vi "Init Hardware.vi"(8 "error in (no error)":errorcluster, 11 "Fluke 1586A Driver in":refnum<class "Fluke 1586A Driver.lvclass">) -> (0 "error out":errorcluster, 3 "Fluke 1586A Driver out":refnum<class "Fluke 1586A Driver.lvclass">)   [LabVIEW 2024, in "Fluke 1586A Driver.lvclass"]
uses:
  Fluke 1586A Driver.lvclass
  Instrument Driver/Instrument Driver.lvclass/Instrument Driver.ctl
  Fluke 1586A Driver.lvclass/Fluke 1586A Driver.ctl
  VISA Instrument/VISA Instrument.lvclass/VISA Instrument.ctl
  Instrument Driver/Read Recorder name.vi
  Instrument Driver/Write Channel names.vi
  Instrument Driver/Write Channel units.vi
  VISA Instrument/Read VISA resource.vi
  VISA Instrument/Write VISA resource.vi
  GPIB/VISA  Send Receive.vi
  Simple VISA Reader/Simple VISA Reader Driver.lvclass
  File/File Class/File.lvclass
panel:
  out "1st check  Data ready":bool
  out "Buffer content":string[](array[string])
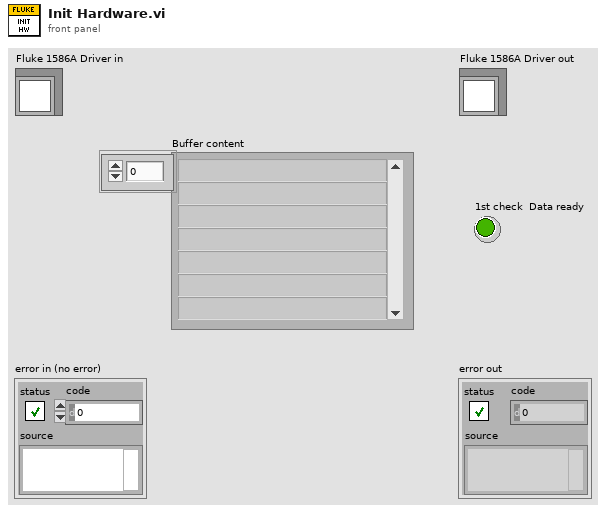
[diagram p1: front panel]
types:
  T1 = typedef "Fluke Configuration.ctl" = cluster{"Channels":string}
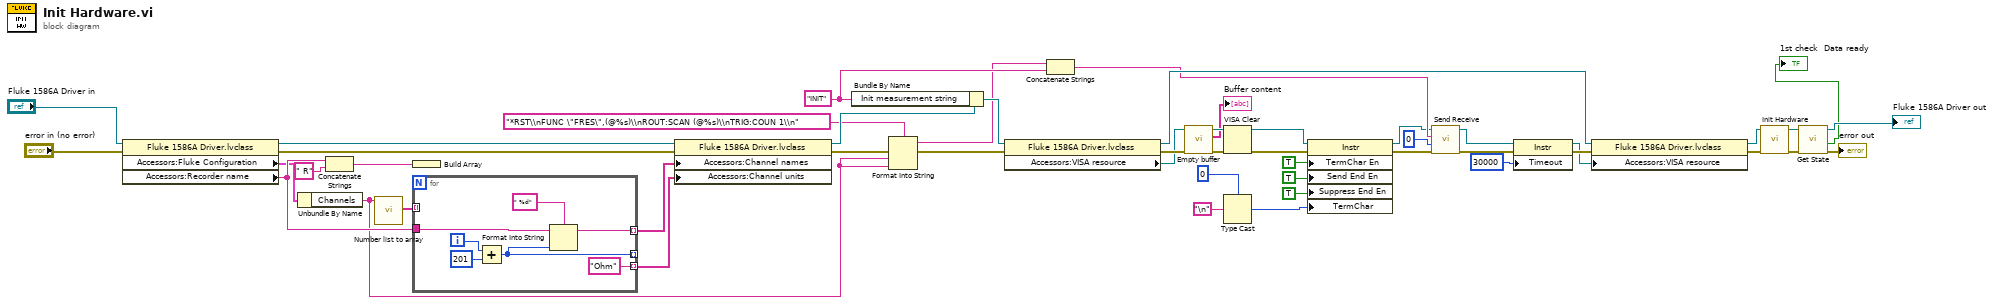
[diagram p0: block diagram]
diagram:
  w34 = "INIT" ("Init measurement string")
  n1 = property class="Fluke 1586A Driver.lvclass"(reference="Fluke 1586A Driver in", error in="error in (no error)") -> (reference out=w47:refnum<class "Fluke 1586A Driver.lvclass">, error out=w48:errorcluster, "Accessors:Fluke Configuration"=w12:T1, "Accessors:Recorder name"=w13:string)
  n2 = Unbundle By Name(w12) -> ("Channels"=w10:string)
  n3 = Concatenate Strings(w13, " R") -> (w49:string)
  n4 = call "Number list to array.vi"("Number list"=w10) -> ("Full names"=w11:string[])  [unwired: 7 in, 3 out]
  n5 = Build Array(w49) -> ()  [unwired: 1 out]
  n6 = for {
    tunnel: [w54] -> _ mode=indexing
    tunnel: w13 -> [w53]
    tunnel: [w51] -> w42 mode=indexing
    tunnel: ["Ohm"] -> w41 mode=indexing
    tunnel: w11 -> [_] mode=indexing
    i -> [w56]
    n7 = Add(x=w56, y=201) -> (x+y=w54:i32)
    n8 = Format Into String(format string=" %d", initial string=w53, w54) -> (resulting string=w51:string)  [unwired: 1 in, 1 out]
  }
  n9 = property class="Fluke 1586A Driver.lvclass"(reference=w47, error in=w48, "Accessors:Channel names"=w42, "Accessors:Channel units"=w41) -> (reference out=w43:refnum<class "Fluke 1586A Driver.lvclass">, error out=w9:errorcluster)
  n10 = Bundle By Name(cluster=w43, "Init measurement string"=w34) -> (w38:refnum<class "Fluke 1586A Driver.lvclass">)
  n11 = Format Into String(format string="*RST\\nFUNC \"FRES\",(@%s)\\nROUT:SCAN (@%s)\\nTRIG:COUN 1\\n" ("string"), error in=w9, w10, w10) -> (resulting string=w6:string, error out=w8:errorcluster)  [unwired: 1 in]
  n12 = property class="Fluke 1586A Driver.lvclass"(reference=w38, error in=w8) -> (reference out=w37:refnum<class "Fluke 1586A Driver.lvclass">, error out=w39:errorcluster, "Accessors:VISA resource"=w16:refnum<visa-resource-name>)
  n13 = Concatenate Strings(w6, w34) -> (w32:string)
  n14 = call "Empty buffer.vi"("Error In"=w39, "VISA resource name"=w16) -> ("Error Out"=w17:errorcluster, "Buffer content"=→"Buffer content":string[], "VISA resource name out"=w15:refnum<visa-resource-name>)  [unwired: 7 in]
  n15 = VISA Clear(VISA resource name=w15, error in (no error)=w17) -> (VISA resource name out=w25:refnum<visa-resource-name>, error out=w24:errorcluster)
  n16 = Type Cast(type=u8 0, x="\n" ("Line Feed Constant")) -> (*(type *) &x=w28:u8)
  n17 = property class="Instr"(reference=w25, error in=w24, "TermChar En"=TRUE ("Message Based Settings:Termination Character Enable"), "Send End En"=TRUE ("Message Based Settings:Send End Enable"), "Suppress End En"=TRUE ("Message Based Settings:Suppress End Enable"), "TermChar"=w28) -> (reference out=w22:refnum<visa-resource-name>, error out=w23:errorcluster)
  n18 = call-poly "Send Receive.vi"("error in (no error)"=w23, "Receive count"=0, "data string in"=w32, "VISA Resource Name"=w22) -> ("error out"=w40:errorcluster, "VISA Resource Name Out"=w20:refnum<visa-resource-name>)  [unwired: 5 in, 1 out]
  n19 = property class="Instr"(reference=w20, error in=w40, "Timeout"=u32 30000 ("General Settings:Timeout Value")) -> (reference out=w19:refnum<visa-resource-name>, error out=w21:errorcluster)
  n20 = property class="Fluke 1586A Driver.lvclass"(reference=w37, error in=w21, "Accessors:VISA resource"=w19) -> (reference out=w36:refnum<class "Fluke 1586A Driver.lvclass">, error out=w35:errorcluster)
  n21 = call-parent "Init Hardware.vi"("error in (no error)"=w35, "Instrument Driver in"=w36) -> ("error out"=w3:errorcluster, "Instrument Driver out"=w5:refnum<class "Fluke 1586A Driver.lvclass">)  [unwired: 8 in]
  n22 = call-dynamic "Get State.vi"("error in (no error)"=w3, "Fluke 1586A Driver in"=w5) -> ("error out"=→"error out":errorcluster, "Data ready"=→"1st check  Data ready":bool, "Fluke 1586A Driver out"=→"Fluke 1586A Driver out":refnum<class "Fluke 1586A Driver.lvclass">)  [unwired: 4 in, 3 out]
